vi "piezoDoubleSyncLearn.vi"() -> ()   [LabVIEW 2017]
uses:
  <vilib>/DAQmx/read.llb/DAQmx Read (Analog 2D DBL NChan NSamp).vi
  <vilib>/DAQmx/read.llb/DAQmx Read (Analog 1D DBL NChan 1Samp).vi
  globalUtilities.vi
  globalDevices.vi
  <vilib>/DAQmx/create/channels.llb/DAQmx Create Channel (AI-Voltage-Basic).vi
  <vilib>/DAQmx/configure/timing.llb/DAQmx Timing (Sample Clock).vi
  <vilib>/DAQmx/miscellaneous.llb/DAQmx Fill In Error Info.vi
panel:
  in  "shift piezo1":dbl=0.5 format="%#_13g"
  in  "acquisitionVolumeHeight":dbl=50.0 format="%#_13g"
  out "x/y":dbl
  in  "shift piezo2":dbl=0.5 format="%#_13g"
  out "adapted functions in piezo1 space":dbl[][](graph)
  out "current positions":cluster{"Waveform":dbl, "Waveform":dbl}(graph)
  in  "stop motion":bool
  out "iteration":i32
  in  "stop":bool
  out "difference between adapted functions":dbl[](graph)
  out "adapted functions":dbl[][](graph)
  out "t0":dbl
  out "original functions":dbl[][](graph)
  # "LEARN HOW TO SYNCHRONIZE PIEZOS WITH DIFFERENT DYNAMICAL PROPERTIES"
  # "EXTRACT BARE DELAY"
  # "LET THE PIEZOS RUN"
  # "LEARN TO ADAPT FUNCTION SET ON PIEZO2 TO MATCH PIEZO1"
  # "Do this in the space of piezo1, i.e. without the conversions for remote focussing."
  # "1 um = 0.05 V\n0.01 V = 200 nm"
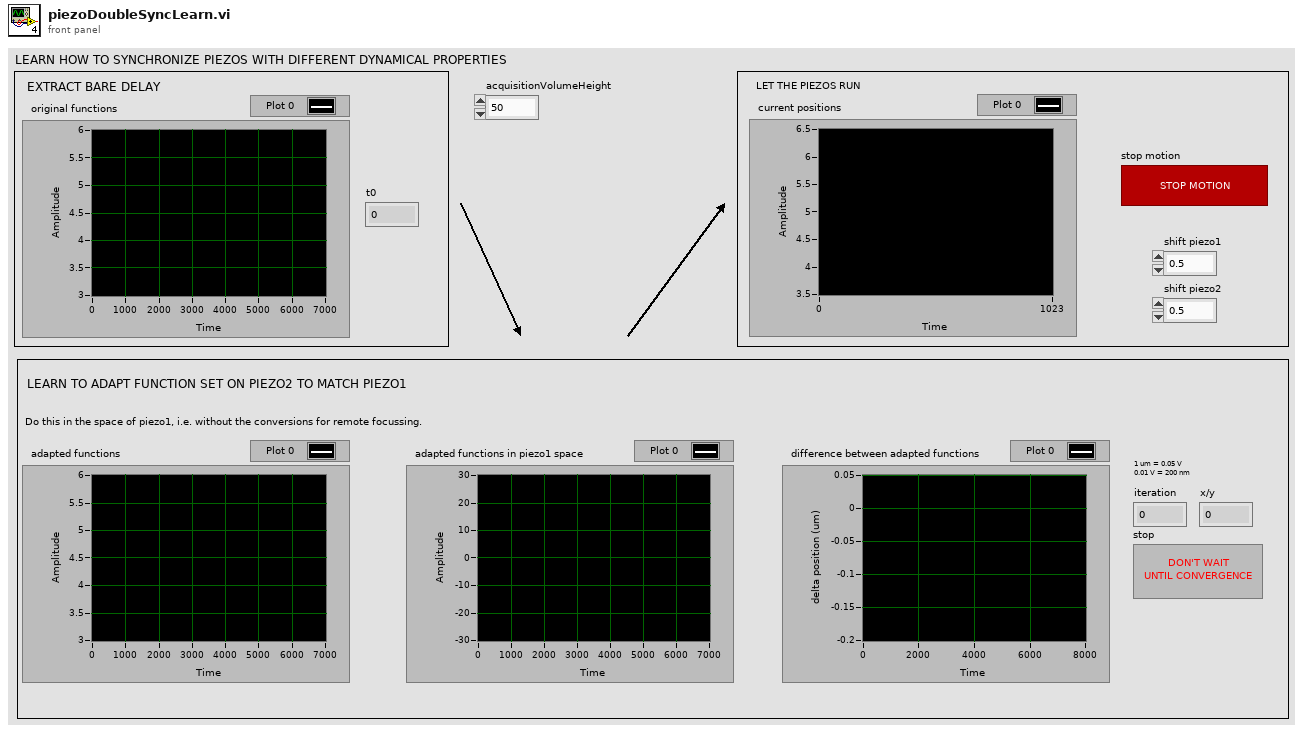
[diagram p1: front panel]
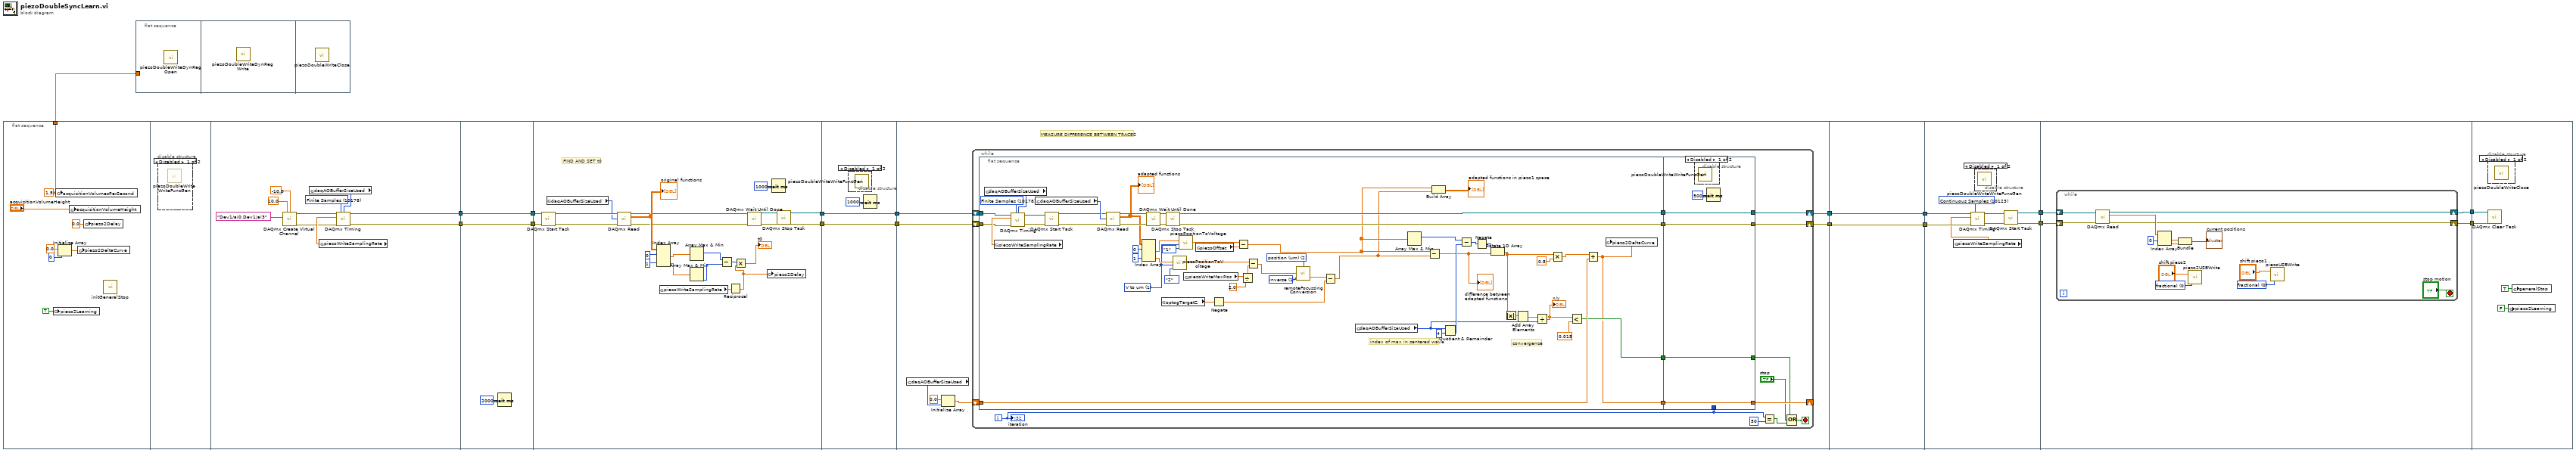
[diagram p0: block diagram]
diagram:
  n1 = flat-sequence {
    tunnel: [w19] -> w1
    tunnel: [w30] -> w15
    tunnel: [w29] -> w14
    tunnel: w14 -> [w37]
    tunnel: [w37] -> w17
    tunnel: w15 -> [w36]
    tunnel: [w36] -> w16
    tunnel: w17 -> [w59]
    tunnel: w16 -> [w60]
    tunnel: [w42] -> w12
    tunnel: [w41] -> w8
    tunnel: [w63] -> w13
    tunnel: w12 -> [w62]
    tunnel: [w62] -> w11
    tunnel: w8 -> [w63]
    tunnel: w13 -> [w67]
    tunnel: w11 -> [w68]
    tunnel: [w70] -> w10
    tunnel: [w69] -> w9
    tunnel: w10 -> [w149]
    tunnel: w9 -> [w148]
    tunnel: [w149] -> w7
    tunnel: [w148] -> w6
    tunnel: w7 -> [w155]
    tunnel: w6 -> [w154]
    tunnel: [w151] -> w5
    tunnel: [w150] -> w4
    tunnel: w5 -> [w161]
    tunnel: w4 -> [w160]
    tunnel: [w159] -> w3
    tunnel: [w158] -> w2
    tunnel: w3 -> [w179]
    tunnel: w2 -> [w178]
    frame #0 {
      w19 = 1.5 ("acquisitionVolumesPerSecond")
      n2 = global write "globalDevices.vi" "piezo2Learning"(TRUE ("piezo2Learning")) -> ()
      n3 = global write "globalUtilities.vi" "acquisitionVolumesPerSecond"(w19) -> ()
      n4 = Initialize Array(0.0 ("element"), 0 ("dimension size")) -> (w21:dbl[])
      n5 = global write "globalUtilities.vi" "acquisitionVolumeHeight"("acquisitionVolumeHeight") -> ()
      n6 = global write "globalDevices.vi" "piezo2DeltaCurve"(w21) -> ()
      n7 = global write "globalDevices.vi" "piezo2Delay"(0.0 ("piezo2Delay")) -> ()
      n8 = call "initGeneralStop.vi"() -> ()  [unwired: 1 in]
    }
    frame #1 {
      n9 = disable-structure shown="Disabled" {
        frame Disabled {
          n10 = call "piezoDoubleWriteWriteFuncGen.vi"() -> ()  [unwired: 1 in, 1 out]
        }
        frame Enabled {
        }
      }
    }
    frame #2 {
      w27 = 10178 items=["Finite Samples"=10178, "Continuous Samples"=10123, "Hardware Timed Single Point"=12522] ("sample mode")
      n11 = call-poly <vilib>:"DAQmx Create Virtual Channel.vi"("maximum value"=10.0, "minimum value"=-10.0, "physical channels"=tag "Dev1/ai0,Dev1/ai3") -> ("task out"=w33:refnum<k21>, "error out"=w31:errorcluster)  [unwired: 11 in]
      n12 = global read "globalDevices.vi" "daqAOBufferSizeUsed"() -> (w26:i32)
      n13 = global read "globalDevices.vi" "piezoWriteSamplingRate"() -> (w32:dbl)
      n14 = call-poly <vilib>:"DAQmx Timing.vi"("task/channels in"=w33, "sample mode"=w27, "samples per channel"=w26, "rate"=w32, "error in"=w31) -> ("task out"=w30:refnum<k21>, "error out"=w29:errorcluster)  [unwired: 9 in]
    }
    frame #3 {
      n15 = Wait (ms)(milliseconds to wait=u32 2000) -> ()  [unwired: 1 out]
    }
    frame #4 {
      # "FIND AND SET t0"
      n16 = call <vilib>:"DAQmx Start Task.vi"("task/channels in"=w60, "error in"=w59) -> ("task out"=w58:refnum<k21>, "error out"=w57:errorcluster)  [unwired: 12 in]
      n17 = global read "globalDevices.vi" "daqAOBufferSizeUsed"() -> (w56:i32)
      n18 = call-poly <vilib>:"DAQmx Read.vi"("task/channels in"=w58, "number of samples per channel"=w56, "error in"=w57) -> ("task out"=w46:refnum<k21>, "data"=w55:dbl[][], "error out"=w45:errorcluster)  [unwired: 10 in]
      "original functions" <- w55
      n19 = Index Array(array=w55, index (row) #1=0 ("index (row)"), index (row) #2=1 ("index (row)")) -> (element #1=w53:dbl[], element #2=w52:dbl[])  [unwired: 2 in]
      n20 = global read "globalDevices.vi" "piezoWriteSamplingRate"() -> (w49:dbl)
      n21 = Array Max & Min(array=w52) -> (min index (indices)=w39:i32)  [unwired: 3 out]
      n22 = Array Max & Min(array=w53) -> (max index (indices)=w51:i32)  [unwired: 3 out]
      n23 = Subtract(x=w51, y=w39) -> (x-y=w50:i32)
      n24 = Reciprocal(x=w49) -> (1/x=w38:dbl)
      n25 = Multiply(x=w50, y=w38) -> (x*y=→"t0":dbl)
      n26 = call <vilib>:"DAQmx Wait Until Done.vi"("task/channels in"=w46, "error in"=w45) -> ("task out"=w44:refnum<k21>, "error out"=w43:errorcluster)  [unwired: 12 in]
      n27 = global write "globalDevices.vi" "piezo2Delay"(w38) -> ()
      n28 = Wait (ms)(milliseconds to wait=u32 1000) -> ()  [unwired: 1 out]
      n29 = call <vilib>:"DAQmx Stop Task.vi"("task/channels in"=w44, "error in"=w43) -> ("task out"=w42:refnum<k21>, "error out"=w41:errorcluster)  [unwired: 12 in]
    }
    frame #5 {
      n30 = disable-structure shown="Disabled" {
        frame Disabled {
          n31 = call "piezoDoubleWriteWriteFuncGen.vi"() -> ()  [unwired: 1 in, 1 out]
        }
        frame Enabled {
        }
      }
      n32 = Wait (ms)(milliseconds to wait=u32 1000) -> ()  [unwired: 1 out]
    }
    frame #6 {
      # "MEASURE DIFFERENCE BETWEEN TRACES"
      n33 = global read "globalDevices.vi" "daqAOBufferSizeUsed"() -> (w65:i32)
      n34 = Initialize Array(0.0 ("element"), w65) -> (w64:dbl[])
      n35 = while {
        shift-right: [w84] -> w70
        shift-left: w68 -> [w86]
        shift-right: [w83] -> w69
        shift-left: w67 -> [w85]
        shift-right: [w82] -> _
        shift-left: w64 -> [w81]
        i -> [w73]
        stop <- w74 stop-if-true
        n36 = flat-sequence {
          tunnel: w86 -> [w134]
          tunnel: w85 -> [w133]
          tunnel: w81 -> [w123]
          tunnel: [w125] -> w80
          tunnel: [w124] -> w79
          tunnel: [w90] -> w78
          tunnel: [w114] -> w77
          tunnel: [w145] -> w82
          tunnel: [w146] -> w83
          tunnel: [w147] -> w84
          tunnel: w80 -> [w147]
          tunnel: w79 -> [w146]
          tunnel: w78 -> [w145]
          tunnel: [w143] -> w75
          tunnel: w77 -> [w143]
          tunnel: w73 -> [_]
          frame #0 {
            w104 = u16 1 items=["um to V", "V to um"] ("mode")
            w108 = u16 2 items=["fractional", "voltage (V)", "position (um)"] ("units")
            w109 = u16 1 items=["direct", "inverse"] ("mode")
            w136 = 10178 items=["Finite Samples"=10178, "Continuous Samples"=10123, "Hardware Timed Single Point"=12522] ("sample mode")
            # "convergence"
            # "index of max in centered wave"
            n37 = global read "globalDevices.vi" "daqAOBufferSizeUsed"() -> (w135:i32)
            n38 = global read "globalDevices.vi" "piezoWriteSamplingRate"() -> (w137:dbl)
            n39 = call-poly <vilib>:"DAQmx Timing.vi"("task/channels in"=w134, "sample mode"=w136, "samples per channel"=w135, "rate"=w137, "error in"=w133) -> ("task out"=w132:refnum<k21>, "error out"=w131:errorcluster)  [unwired: 9 in]
            n40 = global read "globalDevices.vi" "daqAOBufferSizeUsed"() -> (w142:i32)
            n41 = call <vilib>:"DAQmx Start Task.vi"("task/channels in"=w132, "error in"=w131) -> ("task out"=w141:refnum<k21>, "error out"=w140:errorcluster)  [unwired: 12 in]
            n42 = call-poly <vilib>:"DAQmx Read.vi"("task/channels in"=w141, "number of samples per channel"=w142, "error in"=w140) -> ("task out"=w139:refnum<k21>, "data"=w130:dbl[][], "error out"=w138:errorcluster)  [unwired: 10 in]
            "adapted functions" <- w130
            n43 = Index Array(array=w130, index (row) #1=0 ("index (row)"), index (row) #2=1 ("index (row)")) -> (element #1=w107:dbl[], element #2=w105:dbl[])  [unwired: 2 in]
            n44 = call <vilib>:"DAQmx Wait Until Done.vi"("task/channels in"=w139, "error in"=w138) -> ("task out"=w127:refnum<k21>, "error out"=w126:errorcluster)  [unwired: 12 in]
            n45 = global read "globalUtilities.vi" "optogTargetZ"() -> (w99:dbl)
            n46 = call <vilib>:"DAQmx Stop Task.vi"("task/channels in"=w127, "error in"=w126) -> ("task out"=w125:refnum<k21>, "error out"=w124:errorcluster)  [unwired: 12 in]
            n47 = call "piezoPositionToVoltage.vi"("piezo"=enum16{"1", "2"}."2", "mode"=w104, "in (array)"=w105) -> ("out (array)"=w95:dbl[])  [unwired: 3 in, 1 out]
            n48 = call "piezoPositionToVoltage.vi"("piezo"=enum16{"1", "2"}."1", "mode"=w104, "in (array)"=w107) -> ("out (array)"=w102:dbl[])  [unwired: 3 in, 1 out]
            n49 = global read "globalDevices.vi" "piezoWriteMaxPos"() -> (w93:dbl)
            n50 = global read "globalUtilities.vi" "piezoOffset"() -> (w101:dbl)
            n51 = Negate(x=w99) -> (-x=w97:dbl)
            n52 = Subtract(x=w102, y=w101) -> (x-y=w100:dbl[])
            n53 = Divide(x=w93, y=2.0) -> (x/y=w94:dbl)
            n54 = Subtract(x=w95, y=w94) -> (x-y=w98:dbl[])
            n55 = call "remoteFocussingConversion.vi"("units"=w108, "mode"=w109, "dz array"=w98) -> ("dz array out"=w96:dbl[])  [unwired: 1 in, 1 out]
            n56 = Subtract(x=w96, y=w97) -> (x-y=w91:dbl[])
            n57 = global read "globalDevices.vi" "daqAOBufferSizeUsed"() -> (w112:i32)
            n58 = Array Max & Min(array=w100) -> (max index (indices)=w121:i32)  [unwired: 3 out]
            n59 = Subtract(x=w100, y=w91) -> (x-y=w117:dbl[])
            "difference between adapted functions" <- w117
            n60 = Build Array(w100, w91) -> (→"adapted functions in piezo1 space":dbl[][])
            n61 = Quotient & Remainder(x=w112, y=4) -> (floor(x/y)=w118:i32)  [unwired: 1 out]
            n62 = Subtract(x=w121, y=w118) -> (x-y=w120:i32)
            n63 = Negate(x=w120) -> (-x=w119:i32)
            n64 = Rotate 1D Array(1:w117, 2:w119) -> (0:w89:dbl[])
            n65 = Absolute Value(x=w89) -> (abs(x)=w115:dbl[])
            n66 = Add Array Elements(numeric array=w115) -> (sum=w111:dbl)
            n67 = Divide(x=w111, y=w112) -> (x/y=w110:dbl)
            "x/y" <- w110
            n68 = Multiply(x=w89, y=0.5) -> (x*y=w88:dbl[])
            n69 = Less?(x=w110, y=0.015) -> (x < y?=w114:bool)
            n70 = Add(x=w88, y=w123) -> (x+y=w90:dbl[])
            n71 = global write "globalDevices.vi" "piezo2DeltaCurve"(w90) -> ()
          }
          frame #1 {
            n72 = disable-structure shown="Disabled" {
              frame Disabled {
                n73 = call "piezoDoubleWriteWriteFuncGen.vi"() -> ()  [unwired: 1 in, 1 out]
              }
              frame Enabled {
              }
            }
            n74 = Wait (ms)(milliseconds to wait=u32 500) -> ()  [unwired: 1 out]
          }
        }
        n75 = Equal?(x=w73, y=50) -> (x = y?=w71:bool)
        n76 = Compound Arithmetic op=OR(w75, "stop", w71) -> (w74:bool)
        "iteration" <- w73
      }
    }
    frame #7 {
    }
    frame #8 {
      w152 = 10123 items=["Finite Samples"=10178, "Continuous Samples"=10123, "Hardware Timed Single Point"=12522] ("sample mode")
      n77 = global read "globalDevices.vi" "piezoWriteSamplingRate"() -> (w153:dbl)
      n78 = call-poly <vilib>:"DAQmx Timing.vi"("task/channels in"=w155, "sample mode"=w152, "rate"=w153, "error in"=w154) -> ("task out"=w156:refnum<k21>, "error out"=w157:errorcluster)  [unwired: 10 in]
      n79 = disable-structure shown="Disabled" {
        frame Disabled {
          n80 = call "piezoDoubleWriteWriteFuncGen.vi"() -> ()  [unwired: 1 in, 1 out]
        }
        frame Enabled {
        }
      }
      n81 = call <vilib>:"DAQmx Start Task.vi"("task/channels in"=w156, "error in"=w157) -> ("task out"=w151:refnum<k21>, "error out"=w150:errorcluster)  [unwired: 12 in]
    }
    frame #9 {
      n82 = while {
        shift-right: [w166] -> w159
        shift-left: w161 -> [w174]
        shift-right: [w167] -> w158
        shift-left: w160 -> [w173]
        stop <- "stop motion" stop-if-true
        w162 = u16 0 items=["fractional", "voltage (V)", "position (um)"] ("mode")
        w163 = u16 0 items=["fractional", "voltage (V)", "position (um)"] ("mode")
        n83 = call-poly <vilib>:"DAQmx Read.vi"("task/channels in"=w174, "error in"=w173) -> ("task out"=w166:refnum<k21>, "data"=w172:dbl[], "error out"=w167:errorcluster)  [unwired: 11 in]
        n84 = Index Array(array=w172, index #1=0 ("index")) -> (element #1=w170:dbl, element #2=w169:dbl)  [unwired: 1 in]
        n85 = Bundle("Waveform"=w170, "Waveform"=w169) -> (→"current positions":cluster{"Waveform":dbl, "Waveform":dbl})  [unwired: 1 in]
        n86 = call "piezo2USBWrite.vi"("mode"=w162, "position"="shift piezo2") -> ()  [unwired: 1 in]
        n87 = call "piezoUSBWrite.vi"("mode"=w163, "position"="shift piezo1") -> ()  [unwired: 1 in]
      }
    }
    frame #10 {
      n88 = call <vilib>:"DAQmx Clear Task.vi"("task in"=w179, "error in"=w178) -> ()  [unwired: 13 in, 1 out]
      n89 = disable-structure shown="Disabled" {
        frame Disabled {
          n90 = call "piezoDoubleWriteClose.vi"() -> ()  [unwired: 1 in]
        }
        frame Enabled {
        }
      }
      n91 = global write "globalDevices.vi" "piezo2Learning"(FALSE ("piezo2Learning")) -> ()
      n92 = global write "globalUtilities.vi" "generalStop"(TRUE ("generalStop")) -> ()
    }
  }
  n93 = flat-sequence {
    tunnel: w1 -> [_]
    frame #0 {
      n94 = call "piezoDoubleWriteDynRegOpen.vi"() -> ()  [unwired: 12 in]
    }
    frame #1 {
      n95 = call "piezoDoubleWriteDynRegWrite.vi"() -> ()  [unwired: 12 in]
    }
    frame #2 {
      n96 = call "piezoDoubleWriteClose.vi"() -> ()  [unwired: 1 in]
    }
  }
